vi "Configure Tare.vi"(8 "error in (no error)":errorcluster, 9 "Preset Tare  (10.0 g)":dbl=10.0 format="%.3f", 10 "Tare (0: Current Weight)":u16(ring) items=["Current Weight", "Preset Value", "Clear Tare"], 11 "VISA resource name":refnum<visa-resource-name>) -> (0 "error out":errorcluster, 3 "VISA resource name out":refnum<visa-resource-name>)   [LabVIEW 2015, in "Ohaus AV Series.lvlib"]
doc: "This VI tares the balance with current or given preset weight. It will also clear any current tare."
uses:
  Ohaus AV Series.lvlib
panel:
  # "grams"
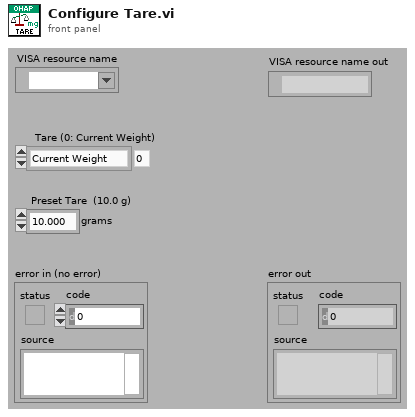
[diagram p1: front panel]
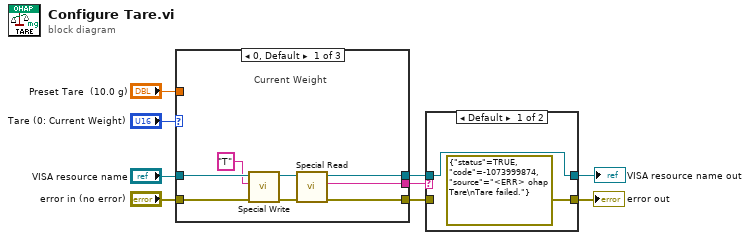
[diagram p0: block diagram]
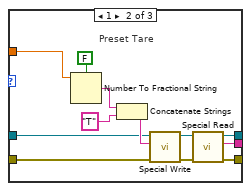
[diagram p3: hidden frame]
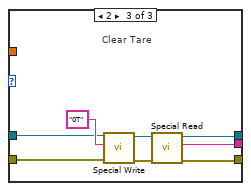
[diagram p4: hidden frame]
diagram:
  n1 = case shown="0, Default" "Tare (0: Current Weight)" {
    tunnel: [w15 w21 w32] -> w6
    tunnel: "VISA resource name" -> [w11 w24 w35]
    tunnel: "error in (no error)" -> [w12 w23 w34]
    tunnel: [w14 w20 w31] -> w5
    tunnel: [w13 w22 w33] -> w4
    tunnel: "Preset Tare  (10.0 g)" -> [_ w19 _]
    frame 0, Default {
      # "Current Weight"
      n2 = call "Special Write.vi"("error in (no error)"=w12, "Input String"="T", "VISA resource name"=w11) -> ("error out"=w16:errorcluster, "VISA resource name out"=w17:refnum<visa-resource-name>)  [unwired: 7 in]
      n3 = call "Special Read.vi"("error in (no error)"=w16, "VISA resource name"=w17) -> ("error out"=w13:errorcluster, "Output String"=w15:string, "VISA resource name out"=w14:refnum<visa-resource-name>)  [unwired: 7 in]
    }
    frame 1 {
      # "Preset Tare"
      n4 = Number To Fractional String(use system decimal point (T)=FALSE, number=w19) -> (F-format string=w28:string)  [unwired: 2 in]
      n5 = Concatenate Strings(w28, "T") -> (w25:string)
      n6 = call "Special Write.vi"("error in (no error)"=w23, "Input String"=w25, "VISA resource name"=w24) -> ("error out"=w26:errorcluster, "VISA resource name out"=w27:refnum<visa-resource-name>)  [unwired: 7 in]
      n7 = call "Special Read.vi"("error in (no error)"=w26, "VISA resource name"=w27) -> ("error out"=w22:errorcluster, "Output String"=w21:string, "VISA resource name out"=w20:refnum<visa-resource-name>)  [unwired: 7 in]
    }
    frame 2 {
      # "Clear Tare"
      n8 = call "Special Write.vi"("error in (no error)"=w34, "Input String"="0T", "VISA resource name"=w35) -> ("error out"=w37:errorcluster, "VISA resource name out"=w30:refnum<visa-resource-name>)  [unwired: 7 in]
      n9 = call "Special Read.vi"("error in (no error)"=w37, "VISA resource name"=w30) -> ("error out"=w33:errorcluster, "Output String"=w32:string, "VISA resource name out"=w31:refnum<visa-resource-name>)  [unwired: 7 in]
    }
  }
  n10 = case shown="Default" w6 {
    tunnel: [errorcluster {"status"=TRUE, "code"=-1073999874, "source"="<ERR> ohap Tare\nTare failed."} ("error out") w41] -> w3
    tunnel: w5 -> [w38 w40]
    tunnel: w4 -> [_ w41]
    tunnel: [w38 w40] -> w2
    frame Default {
    }
    frame "OK!\r\n" {
    }
  }
  "error out" <- w3
  "VISA resource name out" <- w2
